vi "GetMaxTstDist.vi"(8 "错误输入（无错误）":errorcluster, 11 "当前通道序号":u8) -> (0 "错误输出":errorcluster, 3 "返回值":sgl)   [LabVIEW 2014]
uses:
  X86Dll/ZXUTConfigMgr.dll
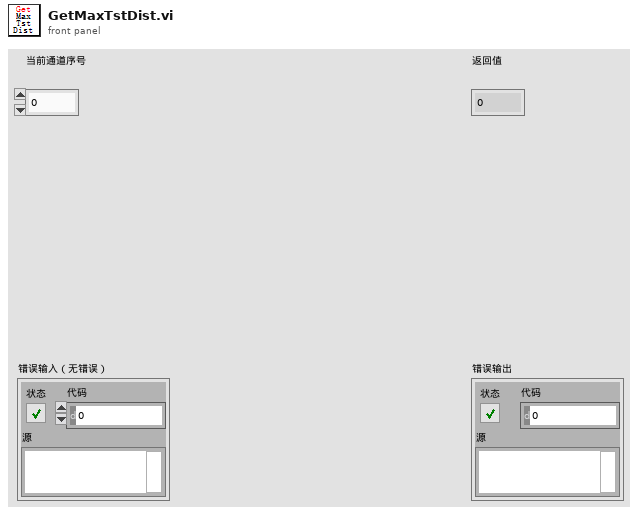
[diagram p1: front panel]
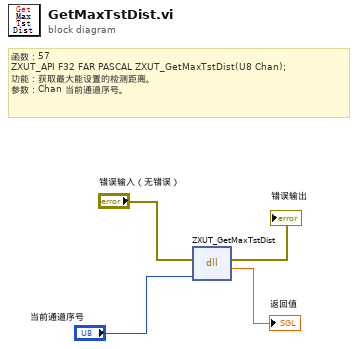
[diagram p0: block diagram]
diagram:
  # "函数：57\nZXUT_API F32\tFAR PASCAL ZXUT_GetMaxTstDist(U8 Chan);\n功能：获取最大能设置的检测距离。\n参数：Chan 当前通道序号。"
  n1 = dll-call lib="D:/Software/Utrasonic on-line monitoring/X86Dll/ZXUTConfigMgr.dll" fn="ZXUT_GetMaxTstDist"(error in="错误输入（无错误）", "Chan"="当前通道序号") -> (error out=→"错误输出":errorcluster, "返回值"=→"返回值":sgl)  [unwired: 3 in, 1 out]
